vi "cutHeader.vi"(10 "element":u32 format="%032b") -> (2 "elementwithoutHeader":u32)   [LabVIEW 2014]
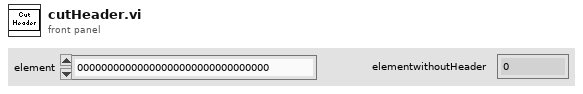
[diagram p1: front panel]
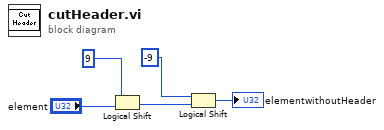
[diagram p0: block diagram]
diagram:
  n1 = Logical Shift(y=i16 9, x="element") -> (x << y=w4:u32)
  n2 = Logical Shift(y=i16 -9, x=w4) -> (x << y=→"elementwithoutHeader":u32)
